vi "Multirecord Acquisition (FPGA)_20221208.vi"() -> ()   [LabVIEW 2021]
doc: "Use this VI as a template for the reconfigurable oscilloscope acquisition design. The block diagram is divided into three main loops.\n\nRegister Bus: This loop initializes the registers that are needed to support the configuration of the device. The FIFO bus, on the left, allows all the other design libraries to communicate with one another. This loop is very important to support the proper behavior of the instrument design library components.\n\nAcquisition: Acquires data from the I/O channels and writes the data into the record memory using the <B>Write</B> VI of the Multirecord Acquisition instrument design library. This VI also evaluates the various acquisition triggers and decides whether to acquire each data value in record memory. The host level VI (Fetch Record.vi) can read acquired records from the DRAM. The data is stored in 2 DRAM banks, each with 768 MB of storage.\n\nFetch: The recorded data is retrieved when the <B>Fetch Single Record</B> VI is run from the host VI. The <B>Write to Fetch DMA FIFO</B> VI writes data to the acq.fetch fifo 0 to transmit record data form the FPGA to the record fetch VIs on the host. This DMA FIFO must have a predefined name based on the instance parameter. By default, it is 0 (since the associated terminal on the <B>Create Resources DRAM Write Read</B> VI is unwired), so the connected FIFO is named acq.fetch fifo 0."
uses:
  FPGA Interface Typedefinitions/Trigger Combination Type.ctl
  <instrlib>/_niInstr/Data Trigger/v1/Shared/Public/Level Configuration FXP(+-,18,1).ctl
  <instrlib>/_niInstr/Data Trigger/v1/Shared/Public/Level Configuration Trigger When.ctl
  <vilib>/Platform/TimedLoop/XDataNode/timing_clust.ctl
  <vilib>/Platform/TimedLoop/XDataNode/nitl_modes.ctl
  <vilib>/Platform/TimedLoop/XDataNode/wakeup.ctl
  <instrlib>/_niInstr/FIFO Register Bus/v1/FPGA/niInstr FIFO Register Bus v1 FPGA.lvclass
  C:/Program Files (x86)/National Instruments/LabVIEW 2021/instr.lib/_niInstr/Instruction Framework/v1/FPGA/Interfaces/Instruction Producer/Instruction Producer.lvclass
  <instrlib>/_niInstr/Multirecord Acquisition/Common/v1/FPGA/niInstr Multirecord Acquisition Common v1 FPGA.lvclass
  C:/Program Files (x86)/National Instruments/LabVIEW 2021/instr.lib/_niInstr/Multirecord Acquisition/Interface/v1/FPGA/niInstr Multirecord Acquisition v1 FPGA.lvclass
  <vilib>/rvi/Emulation/niFpgaSctlEmulationGetInTimedLoop.vi
  <vilib>/rvi/Emulation/niFpgaEmulationReportErrorSimple.vi
  <vilib>/rvi/Emulation/niFpgaGetClockAttributes.vi
  <vilib>/rvi/Emulation/niFpgaCriticalErrorInLSC.vi
  <instrlib>/_niInstr/Multirecord Acquisition/Common/v1/FPGA/Private/Create Fetch DMA FIFO Resources U8x32.vi
  <instrlib>/_niInstr/Multirecord Acquisition/Common/v1/FPGA/Private/Create Resources DRAM U384x2 U768 Write Read.vi
  <instrlib>/_niInstr/Multirecord Acquisition/Interface/v1/FPGA/Private/Retrieve Record U16 Wrapper.vi
  <instrlib>/_niInstr/Multirecord Acquisition/Interface/v1/FPGA/Private/Write to Fetch DMA FIFO U16 Wrapper.vi
  <vilib>/rvi/eio/common/nirviEmuTemplateMethod_errors.vi
  <instrlib>/HSAI-RIO/Config/Group A/v1/FPGA/Digital Correction/Validate 8 Channel Data.vi
  <instrlib>/HSAI-RIO/Config/Group A/v1/FPGA/Digital Correction/Digital Correction (8 Ch).vi
  <instrlib>/HSAI-RIO/Config/Group A/v1/FPGA/Digital Correction/FIR Filter (8 Ch).vi
  DSP/SubVIs/Integer decimationx8ch.vi
  Data Type Conversion/SubVIs/Remove Overflow FXP(+-,18,1)x8ch.vi
  <instrlib>/_niInstr/Channel/v1/FPGA/Private/Select/Select FXP(+-,18,1,)xNspcx8ch.vi
  Trigger/Trigger FXP(+,-,18,1).vi
  Data Type Conversion/SubVIs/Data Type Conversion FXP(+-,18,1) to I16x8ch.vi
  <instrlib>/_niInstr/Channel/v1/FPGA/Private/Select and Interleave/Select And Interleave I16xNspcx8ch.vi
  <instrlib>/_niInstr/Multirecord Acquisition/Interface/v1/FPGA/Private/Write I16 Wrapper.vi
  <vilib>/Platform/TimedLoop/XDataNode/XDataNode.xnode
  <vilib>/eio/EIONode/EIONode.xnode
  <instrlib>/_niInstr/Instruction Framework/v1/FPGA/Top Level Bus/Register Configuration/Register Configuration.lvclass
  <vilib>/Platform/TimedLoop/XDataNode/XDNodeRunTimeDep.lvlib
  <instrlib>/_niInstr/Multirecord Acquisition/Interface/v1/FPGA/niInstr Multirecord Acquisition v1 FPGA.lvclass
  <vilib>/rvi/LocalResourceManager/LocalResourceManager.xnode
  <vilib>/rvi/eio/common/nirviEmuReportErrorAndStop.vi
  <vilib>/rvi/DataTransferAndStorage/Container/Common/niFpgaContainerGetUniqueNameForEmu.vi
  <vilib>/rvi/DataTransferAndStorage/Container/Common/niFpgaContainerSetEmuInfo.vi
  <instrlib>/_niInstr/Channel/v1/FPGA/niInstr Channel v1 FPGA.lvlib
  <instrlib>/_niInstr/Basic Elements/v1/FPGA/niInstr Basic Elements v1 FPGA.lvlib
  <instrlib>/HSAI-RIO/Config/Group A/v1/FPGA/Digital Correction/Digital Correction.lvclass
  <instrlib>/HSAI-RIO/Config/Group A/v1/FPGA/Config Registers/Config Registers.lvclass
  <instrlib>/_niInstr/Multirecord Acquisition/Common/v1/FPGA/Private/Create Resources BRAM U384.vi
  Emulation/SubVIs/2 Element Generate Sine Cos Data FXP(+,-,14,1).vi
  <instrlib>/_niInstr/Multirecord Acquisition/Common/v1/FPGA/Private/Create Resources DRAM U384.vi
  <instrlib>/_niInstr/Multirecord Acquisition/Common/v1/FPGA/Private/Create Resources BRAM U768.vi
  C:/Program Files (x86)/National Instruments/LabVIEW 2021/instr.lib/_niInstr/Multirecord Acquisition/Common/v1/FPGA/niInstr Multirecord Acquisition Common v1 FPGA.lvclass
  FPGA Interface Typedefinitions/FPGA Interface Typedefinitions.lvlib
  <instrlib>/_niInstr/Data Trigger/v1/Shared/niInstr Data Trigger v1 Shared.lvlib
panel:
  in  "trig 7":cluster{"Hi":T1, "Lo":T1}
  in  "trig 6":cluster{"Hi":T1, "Lo":T1}
  in  "trig 5":cluster{"Hi":T1, "Lo":T1}
  in  "trig 4":cluster{"Hi":T1, "Lo":T1}
  in  "trig 3":cluster{"Hi":T1, "Lo":T1}
  in  "trig 2":cluster{"Hi":T1, "Lo":T1}
  in  "trig 1":cluster{"Hi":T1, "Lo":T1}
  in  "trig 0":cluster{"Hi":T1, "Lo":T1}
  in  "trigger.rearm delay":u16=2
  in  "start trigger":bool=TRUE
  in  "reset":bool
  in  "trigger.combination type":T3
  out "fifo reg bus data 0":u64
  out "fifo reg bus status 0":u32
  in  "fifo reg bus ctrl 0":u32
  out "overflow":bool
  in  "dsp.decimation factor":u16
  out "overload":bool
  in  "channel.enable mask":u16=65535 format="%.0b"
  in  "channel.number of channels":u8=8
  # "Register Bus Controls"
  # "FPGA"
  # "Acquisition Loop Controls"
  # "DSP"
  # "Trigger"
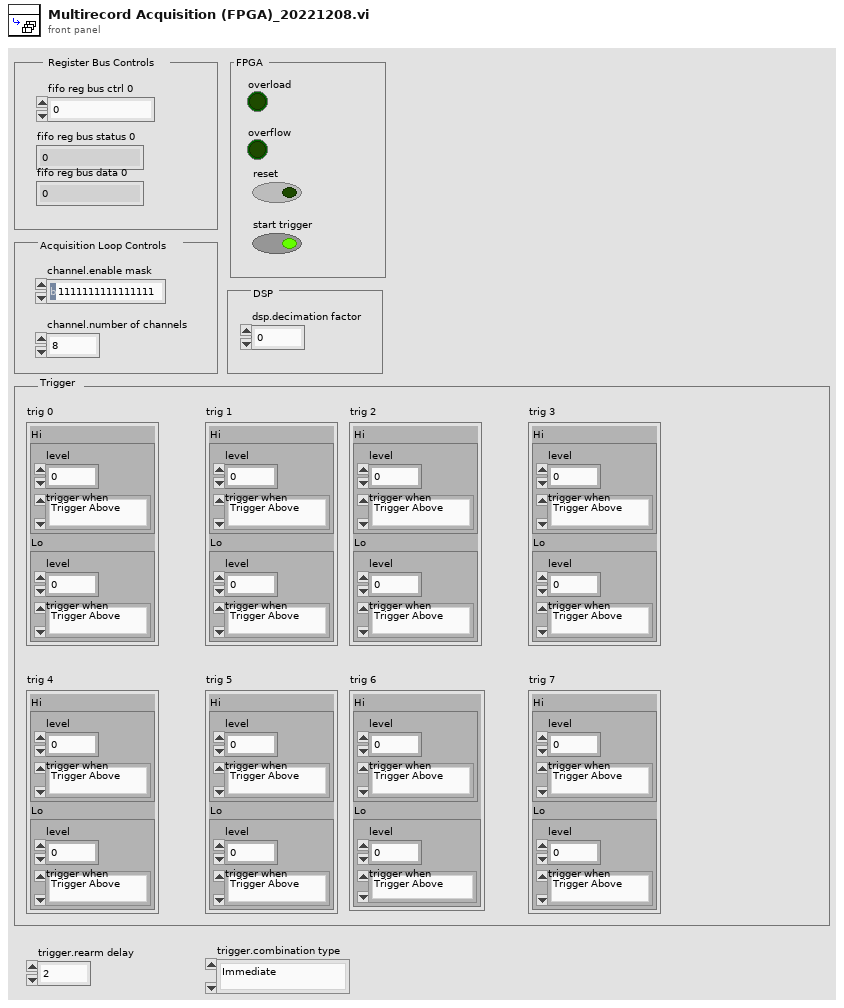
[diagram p1: front panel]
types:
  T1 = typedef "niInstr Data Trigger v1 Shared.lvlib/Level Configuration FXP(+-,18,1).ctl" = cluster{"level":fxp<+/-,18,1>, "trigger when":T2}
  T2 = typedef "niInstr Data Trigger v1 Shared.lvlib/Level Configuration Trigger When.ctl" = enum8{"Trigger Above", "Trigger Below"}
  T3 = typedef "FPGA Interface Typedefinitions.lvlib/Trigger Combination Type.ctl" = enum16{"Immediate", "A", "B", "OR", "AND", "A THEN B", "B THEN A", "High Resolution"}
  T4 = cluster{"memory 1":refnum<k21>, "memory 2":refnum<k21>}
  T5 = typedef "XDNodeRunTimeDep.lvlib/timing_clust.ctl" = cluster{"Expected End [f-1]":u64, "Actual End [f-1]":u64, "Finished Late? [f-1]":bool, "Expected End [i-1]":u64, "Actual End [i-1]":u64, "Finished Late? [i-1]":bool, "Expected Start [i]":u64, "Actual Start [i]":u64, "Expected Start [f]":u64, "Actual Start [f]":u64, "Source Name":string, "Structure Name":string, "Period":i64, "Deadline":i64, "Offset":i64, "Start":i64, "Priority":i32, "Timeout":i32, "Mode":T6, "Wakeup Reason":T7, "Error":errorcluster, "Source Type":string, "Secondary Source Type":string, "Global End Time":u64, "Global Start Time":u64, "Frame Duration":u64, "Iteration Duration":u64, "Assigned CPU":i32, "I/O Scan Engine Mode":u32}
  T6 = typedef "XDNodeRunTimeDep.lvlib/nitl_modes.ctl" = enum32{"No Change", "Process missed periods, maintain original phase", "Discard missed periods, maintain original phase", "Process missed periods, ignore original phase", "Discard missed periods, ignore original phase"}
  T7 = typedef "XDNodeRunTimeDep.lvlib/wakeup.ctl" = enum32{"Normal", "Aborted", "Asynchronous wakeup", "Timing source error", "Timed loop error", "Timeout"}
  T8 = cluster{"Channel 0":fxp<+/-,14,1>[], "Channel 1":fxp<+/-,14,1>[], "Channel 2":fxp<+/-,14,1>[], "Channel 3":fxp<+/-,14,1>[], "Channel 4":fxp<+/-,14,1>[], "Channel 5":fxp<+/-,14,1>[], "Channel 6":fxp<+/-,14,1>[], "Channel 7":fxp<+/-,14,1>[]}
  T9 = cluster{"Channel 0":fxp<+/-,18,1>[], "Channel 1":fxp<+/-,18,1>[], "Channel 2":fxp<+/-,18,1>[], "Channel 3":fxp<+/-,18,1>[], "Channel 4":fxp<+/-,18,1>[], "Channel 5":fxp<+/-,18,1>[], "Channel 6":fxp<+/-,18,1>[], "Channel 7":fxp<+/-,18,1>[]}
  T10 = cluster{"channel 0":fxp<+/-,18,1>[], "channel 1":fxp<+/-,18,1>[], "channel 2":fxp<+/-,18,1>[], "channel 3":fxp<+/-,18,1>[], "channel 4":fxp<+/-,18,1>[], "channel 5":fxp<+/-,18,1>[], "channel 6":fxp<+/-,18,1>[], "channel 7":fxp<+/-,18,1>[]}
  T11 = cluster{"channel 0":i16[], "channel 1":i16[], "channel 2":i16[], "channel 3":i16[], "channel 4":i16[], "channel 5":i16[], "channel 6":i16[], "channel 7":i16[]}
  T12 = typedef "niInstr Multirecord Acquisition v1 FPGA.lvclass/Timestamp.ctl" = cluster{"timestamp":u64, "valid":bool}
  T13 = typedef "niInstr Types v1 Shared.lvlib/Input Triggers.ctl" = cluster{"start":bool, "advance":bool, "reference":bool, "start trigger index":u16, "advance trigger index":u16, "reference trigger index":u16, "reference trigger correction cycle count":u32}
  T14 = typedef "niInstr Types v1 Shared.lvlib/Sample Format.ctl" = cluster{"bits per channel":u16, "samples per clock":u16, "channels":u8}
  T15 = typedef "niInstr Multirecord Acquisition v1 FPGA.lvclass/Events.ctl" = cluster{"ready for start":bool, "ready for advance":bool, "ready for reference":bool, "end of record":bool, "done":bool, "start trigger":bool, "advance trigger":bool, "reference trigger":bool, "start trigger index":u16, "advance trigger index":u16, "reference trigger index":u16}
  T16 = typedef "niInstr Multirecord Acquisition v1 FPGA.lvclass/Retrieve Data Info.ctl" = cluster{"read request size (bits)":u64, "valid data offset (bits)":u16, "valid data size (bits)":u16, "first sample of request":bool, "last sample of request":bool, "Token":T17}
  T17 = typedef "niInstr Types v1 Shared.lvlib/Token.ctl" = cluster{"identifier":u8, "value":u32}
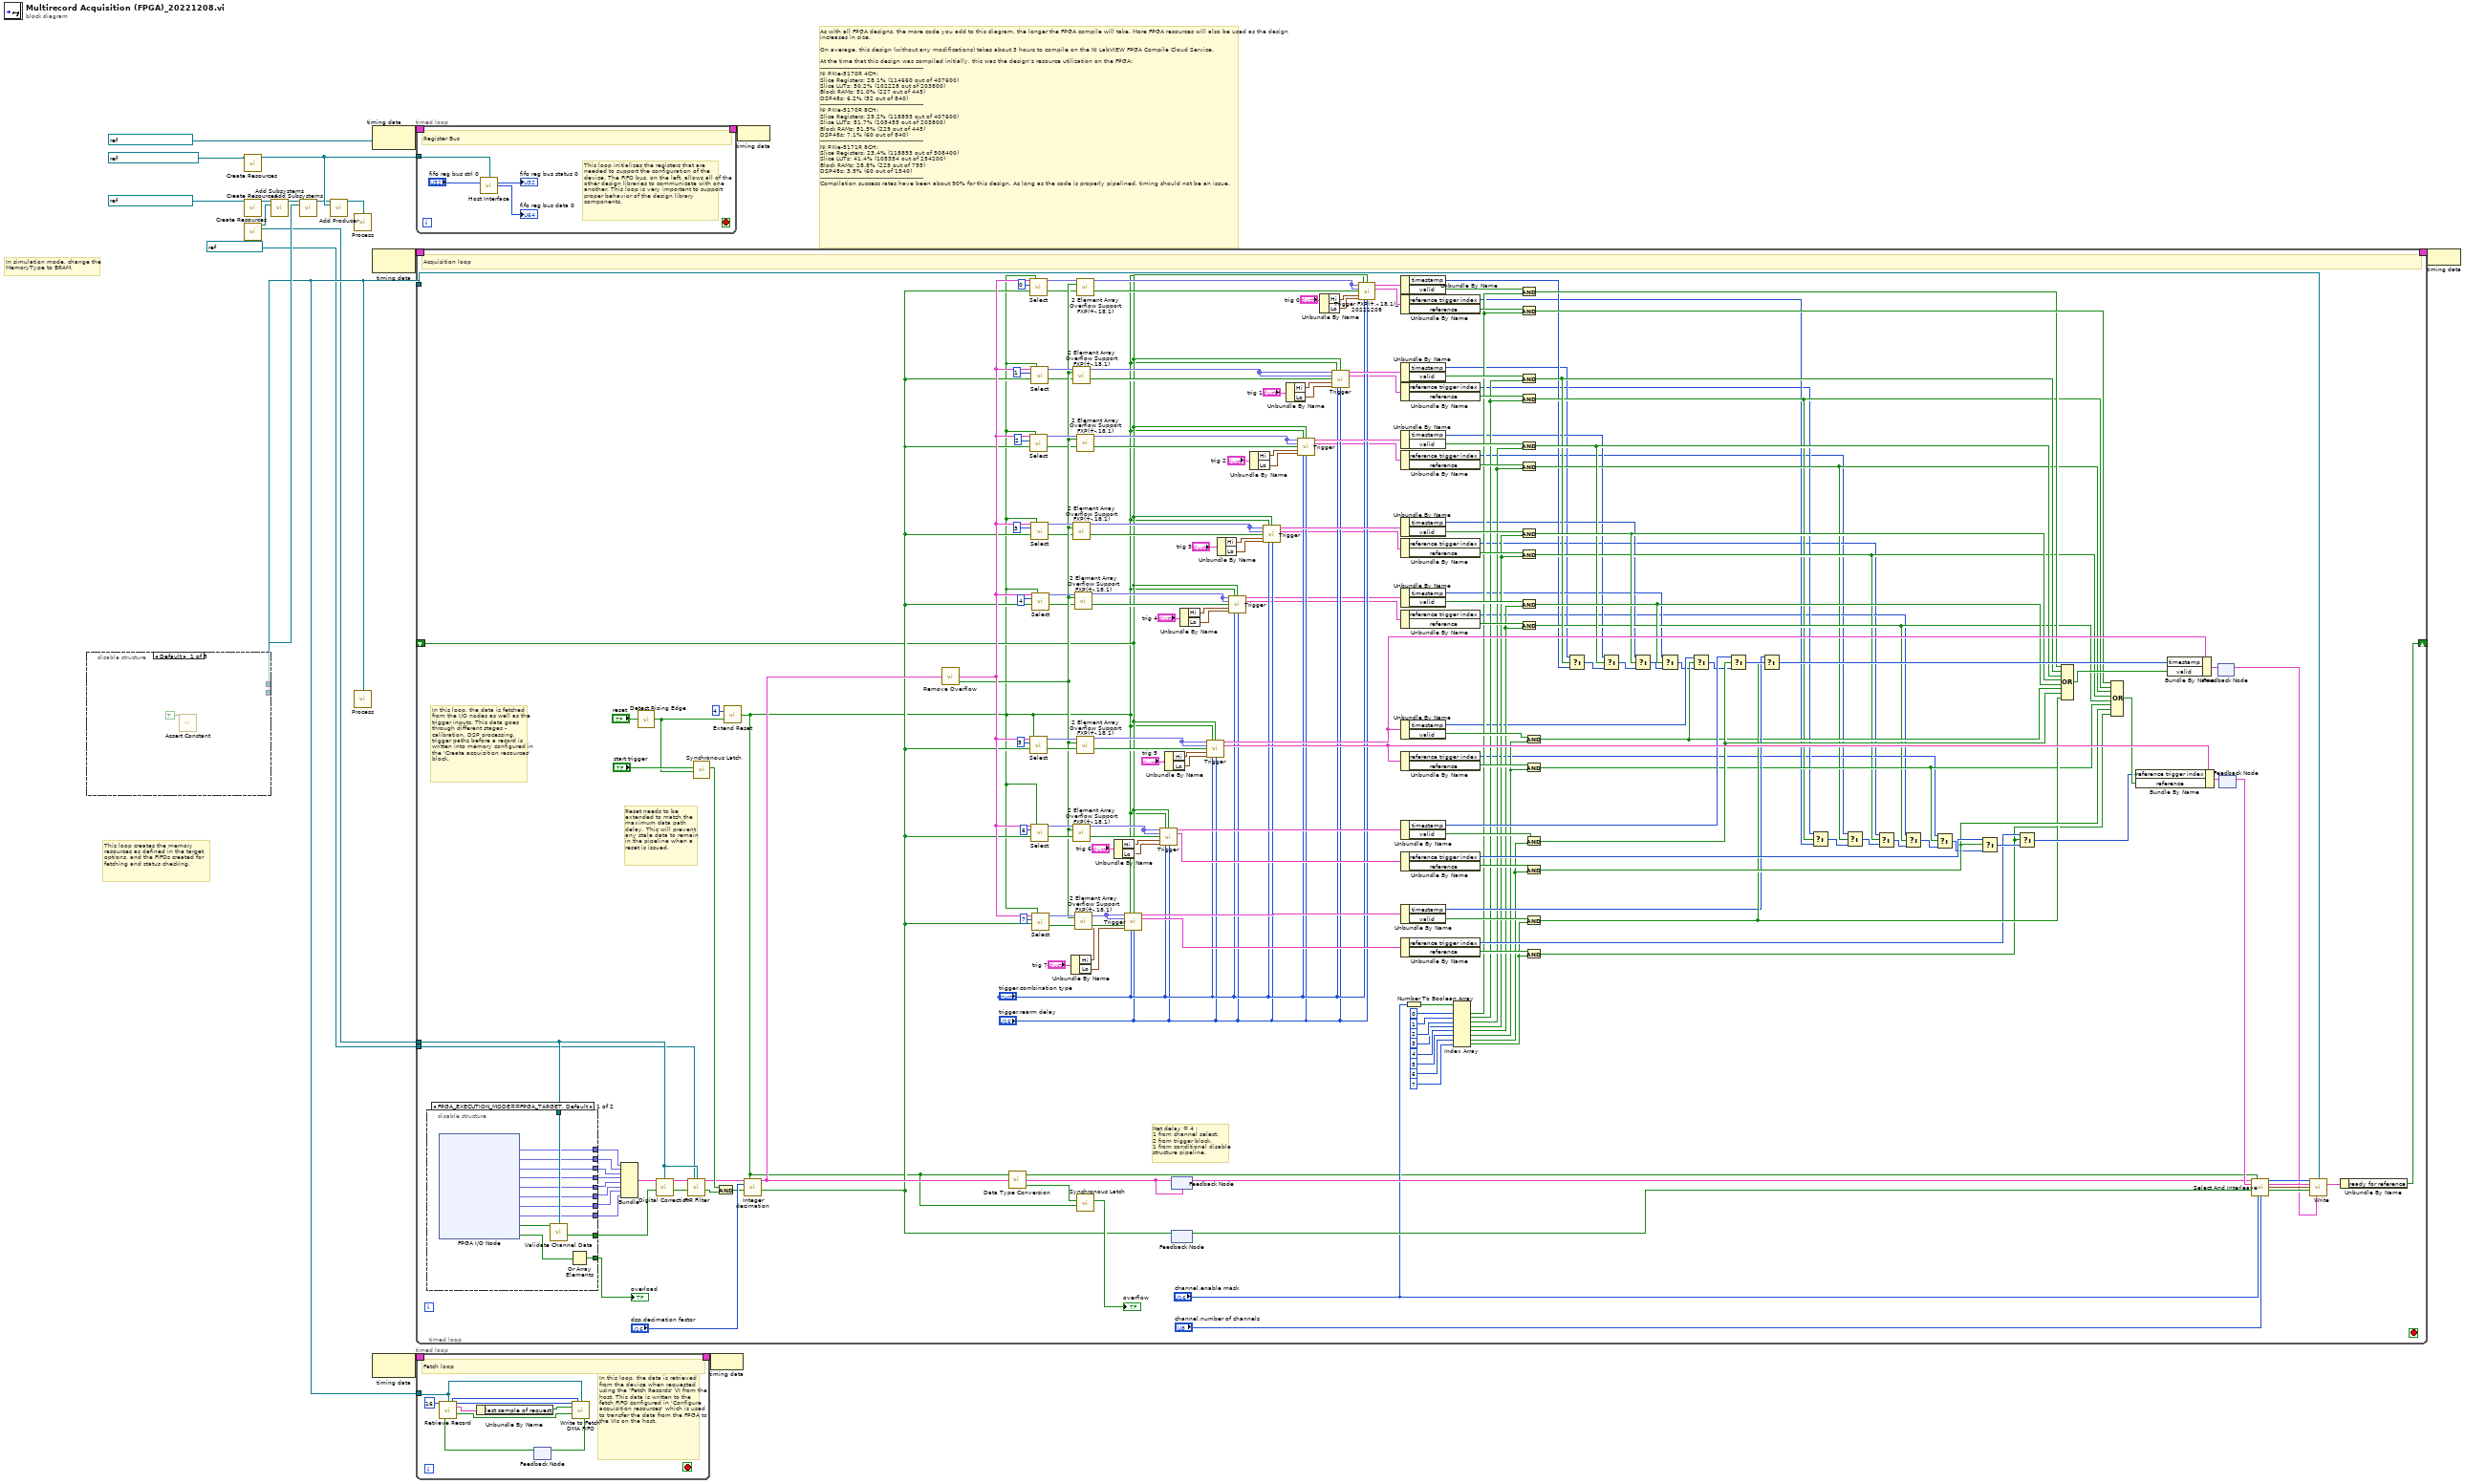
[diagram p0: block diagram]
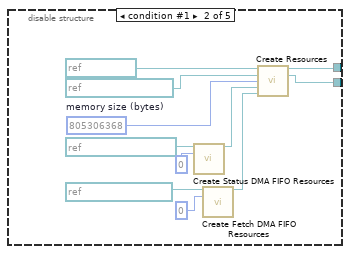
[diagram p2: hidden frame]
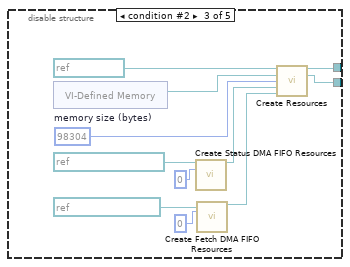
[diagram p3: hidden frame]
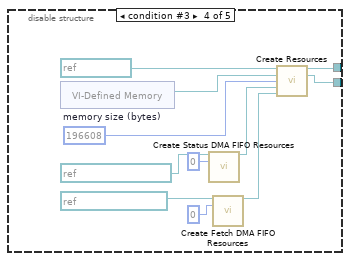
[diagram p4: hidden frame]
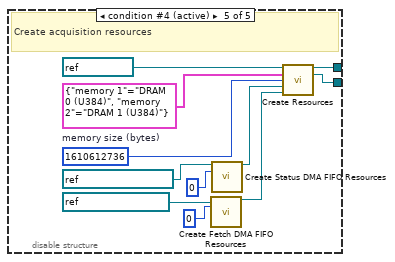
[diagram p5: hidden frame]
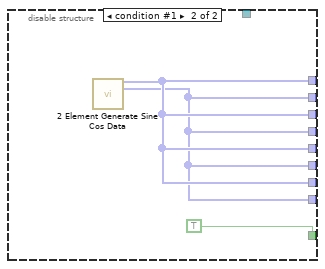
[diagram p6: hidden frame]
diagram:
  # "In simulation mode, change the MemoryType to BRAM."
  # "This loop creates the memory resources as defined in the target options, and the FIFOs created for fetching and status checking."
  # "As with all FPGA designs, the more code you add to this diagram, the longer the FPGA compile will take. More FPGA resources will also be used as the design increases in size.\n\nOn average, this design (without any modifications) takes about 3 hours to compile on the NI LabVIEW FPGA Compile Cloud Service. \n\nAt the time that this design was compiled initially, this was the design's resource utilization on the FPGA:\n------------------------------------------------------\nNI PXIe-5170R 4CH:\nSlice Registers: 28.1% (114660 out of 407600)\nSlice LUTs: 50.2% (102228 out of 203800)\nBlock RAMs: 51.0% (227 out of 445)\nDSP48s: 6.2% (52 out of 840)\n------------------------------------------------------\nNI PXIe-5170R 8CH:\nSlice Registers: 29.2% (118893 out of 407600)\nSlice LUTs: 51.7% (105455 out of 203800)\nBlock RAMs: 51.5% (229 out of 445)\nDSP48s: 7.1% (60 out of 840)\n------------------------------------------------------\nNI PXIe-5171R 8CH:\nSlice Registers: 23.4% (118893 out of 508400)\nSlice LUTs: 41.4% (105354 out of 254200)\nBlock RAMs: 28.8% (229 out of 795)\nDSP48s: 3.9% (60 out of 1540)\n------------------------------------------------------\nCompilation success rates have been about 90% for this design. As long as the code is properly pipelined, timing should not be an issue."
  n1 = disable-structure shown="Default" {
    disable-tunnel: [_ w29 w40 w51 w62] -> w4
    disable-tunnel: [_ w26 w36 w47 w59] -> w7
    frame condition #0 {
      n2 = call <instrlib>:"Assert Constant.vi"("constant terminal"=TRUE) -> ()  [unwired: 15 in]
    }
    frame condition #1 {
      w30 = u64 805306368  # memory size (bytes)
      n3 = call <instrlib>:"Create Status DMA FIFO Resources.vi"("status dma fifo in"=refnum<k21> "acq.status fifo 0" ("status dma fifo"), "fifo instance"=u8 0) -> ("status dma fifo out"=w21:refnum<class "niInstr Status FIFO v1 FPGA.lvclass">)  [unwired: 13 in]
      n4 = call-poly <instrlib>:"Create Fetch DMA FIFO Resources.vi"("fetch dma fifo in"=refnum<k21> "acq.fetch fifo 0", "fifo instance"=u8 0) -> ("fetch dma fifo out"=w27:refnum<class "niInstr Fetch FIFO v1 FPGA.lvclass">)  [unwired: 13 in]
      n5 = call-poly <instrlib>:"Create Resources.vi"("memory clock"=refnum<k21> "160MHz" ("process clock"), "memory"=refnum<k21> "DRAM 0 (U384)" ("dram"), "memory size (bytes)"=w30, "status dma fifo resources"=w21, "fetch dma fifo resources"=w27) -> ("acquisition resources"=w29:refnum<class "niInstr Multirecord Acquisition Common v1 FPGA.lvclass">, "acquisition subsystem"=w26:refnum<class "Address Space Collection.lvclass">)  [unwired: 9 in]
    }
    frame condition #2 {
      w41 = u64 98304  # memory size (bytes)
      n6 = xnode "VI-Defined Memory"() -> ("Memory Out"=w42:refnum<k21>)
      n7 = call <instrlib>:"Create Status DMA FIFO Resources.vi"("status dma fifo in"=refnum<k21> "acq.status fifo 0" ("status dma fifo"), "fifo instance"=u8 0) -> ("status dma fifo out"=w33:refnum<class "niInstr Status FIFO v1 FPGA.lvclass">)  [unwired: 13 in]
      n8 = call-poly <instrlib>:"Create Fetch DMA FIFO Resources.vi"("fetch dma fifo in"=refnum<k21> "acq.fetch fifo 0", "fifo instance"=u8 0) -> ("fetch dma fifo out"=w37:refnum<class "niInstr Fetch FIFO v1 FPGA.lvclass">)  [unwired: 13 in]
      n9 = call-poly <instrlib>:"Create Resources.vi"("memory clock"=refnum<k21> "160MHz" ("process clock"), "memory"=w42, "memory size (bytes)"=w41, "status dma fifo resources"=w33, "fetch dma fifo resources"=w37) -> ("acquisition resources"=w40:refnum<class "niInstr Multirecord Acquisition Common v1 FPGA.lvclass">, "acquisition subsystem"=w36:refnum<class "Address Space Collection.lvclass">)  [unwired: 9 in]
    }
    frame condition #3 {
      w52 = u64 196608  # memory size (bytes)
      n10 = xnode "VI-Defined Memory"() -> ("Memory Out"=w53:refnum<k21>)
      n11 = call <instrlib>:"Create Status DMA FIFO Resources.vi"("status dma fifo in"=refnum<k21> "acq.status fifo 0" ("status dma fifo"), "fifo instance"=u8 0) -> ("status dma fifo out"=w45:refnum<class "niInstr Status FIFO v1 FPGA.lvclass">)  [unwired: 13 in]
      n12 = call-poly <instrlib>:"Create Fetch DMA FIFO Resources.vi"("fetch dma fifo in"=refnum<k21> "acq.fetch fifo 0", "fifo instance"=u8 0) -> ("fetch dma fifo out"=w48:refnum<class "niInstr Fetch FIFO v1 FPGA.lvclass">)  [unwired: 13 in]
      n13 = call-poly <instrlib>:"Create Resources.vi"("memory clock"=refnum<k21> "160MHz" ("process clock"), "memory"=w53, "memory size (bytes)"=w52, "status dma fifo resources"=w45, "fetch dma fifo resources"=w48) -> ("acquisition resources"=w51:refnum<class "niInstr Multirecord Acquisition Common v1 FPGA.lvclass">, "acquisition subsystem"=w47:refnum<class "Address Space Collection.lvclass">)  [unwired: 9 in]
    }
    frame condition #4 (active) {
      w64 = u64 1610612736  # memory size (bytes)
      # "Create acquisition resources"
      n14 = call-poly <instrlib>:"Create Fetch DMA FIFO Resources.vi"("fetch dma fifo in"=refnum<k21> "acq.fetch fifo 0", "fifo instance"=u8 0) -> ("fetch dma fifo out"=w61:refnum<class "niInstr Fetch FIFO v1 FPGA.lvclass">)  [unwired: 13 in]
      n15 = call <instrlib>:"Create Status DMA FIFO Resources.vi"("status dma fifo in"=refnum<k21> "acq.status fifo 0" ("status dma fifo"), "fifo instance"=u8 0) -> ("status dma fifo out"=w56:refnum<class "niInstr Status FIFO v1 FPGA.lvclass">)  [unwired: 13 in]
      n16 = call-poly <instrlib>:"Create Resources.vi"("memory clock"=refnum<k21> "160MHz" ("process clock"), "memory"=T4 {"memory 1"="DRAM 0 (U384)", "memory 2"="DRAM 1 (U384)"}, "memory size (bytes)"=w64, "status dma fifo resources"=w56, "fetch dma fifo resources"=w61) -> ("acquisition resources"=w62:refnum<class "niInstr Multirecord Acquisition Common v1 FPGA.lvclass">, "acquisition subsystem"=w59:refnum<class "Address Space Collection.lvclass">)  [unwired: 9 in]
    }
  }
  n17 = call <instrlib>:"Create Resources.vi"("instruction fifo"=refnum<k21> "reg.host instruction fifo 0" ("FIFO")) -> ("fifo register bus"=w6:refnum<class "niInstr FIFO Register Bus v1 FPGA.lvclass">)  [unwired: 14 in]
  n18 = call <instrlib>:"Create Resources.vi"("register clock"=refnum<k21> "40 MHz Onboard Clock" ("Source Name")) -> ("register configuration"=w10:refnum<class "Register Configuration.lvclass">)  [unwired: 14 in]
  n19 = call <instrlib>:"Create Resources.vi"() -> ("config subsystems"=w8:refnum<class "Address Space Collection.lvclass">, "digital correction resources"=w1:refnum<class "Digital Correction.lvclass">)  [unwired: 14 in]
  n20 = call-dynamic "Add Subsystems.vi"("register configuration in"=w10, "subsystems"=w8) -> ("register configuration out"=w9:refnum<class "Register Configuration.lvclass">)  [unwired: 13 in]
  n21 = call-dynamic "Add Subsystems.vi"("register configuration in"=w9, "subsystems"=w7) -> ("register configuration out"=w3:refnum<class "Register Configuration.lvclass">)  [unwired: 13 in]
  n22 = call-dynamic "Add Producer.vi"("register configuration in"=w3, "instruction producer"=w6) -> ("register configuration out"=w5:refnum<class "Register Configuration.lvclass">)  [unwired: 13 in]
  n23 = call-dynamic "Process.vi"("register configuration"=w5) -> ()  [unwired: 15 in]
  n24 = call-dynamic "Process.vi"("acquisition resources"=w4) -> ()  [unwired: 15 in]
  n25 = node-c288(refnum<k21> "40 MHz Onboard Clock" ("Source Name")) -> (w19:T5)
  n26 = node-c288() -> (w17:T5)  [unwired: 1 in]
  n27 = node-c288() -> (w15:T5)  [unwired: 1 in]
  n28 = timed-loop {
    timing: w19 -> [_]
    timing-out: [_] -> w18
    tunnel: w6 -> [w68]
    stop <- _ stop-if-true
    # "This loop initializes the registers that are needed to support the configuration of the device. The FIFO bus, on the left, allows all of the other design libraries to communicate with one another. This loop is very important to support proper behavior of the design library components."
    # "Register Bus"
    n29 = call <instrlib>:"Host Interface.vi"("fifo register bus"=w68, "fifo reg bus ctrl 0"="fifo reg bus ctrl 0") -> ("fifo reg bus status 0"=→"fifo reg bus status 0":u32, "fifo reg bus data 0"=→"fifo reg bus data 0":u64)  [unwired: 12 in]
  }
  n30 = timed-loop {
    timing: w17 -> [_]
    timing-out: [_] -> w16
    tunnel: w4 -> [w272]
    tunnel: w1 -> [w255]
    shift-right: [w264] -> _
    shift-left: _ -> [w167]
    tunnel: refnum<k21> "Data Clock x2" -> [w252]
    stop <- _ stop-if-true
    # "Net delay = 4 :\n1 from channel select.\n2 from trigger block.\n1 from conditional disable structure pipeline."
    # "Reset needs to be extended to match the maximum data path delay. This will prevent any stale data to remain in the pipeline when a reset is issued."
    # "In this loop, the data is fetched from the I/O nodes as well as the trigger inputs. This data goes through different stages - calibration, DSP processing, trigger paths before a record is written into memory configured in the 'Create acquisition resources' block."
    # "Acquisition loop"
    n31 = disable-structure shown="FPGA_EXECUTION_MODE==FPGA_TARGET, Default" {
      disable-tunnel: [w284 w289] -> w251
      disable-tunnel: [w283 w288] -> w250
      disable-tunnel: [w282 w289] -> w249
      disable-tunnel: [w281 w288] -> w248
      disable-tunnel: [w280 w289] -> w247
      disable-tunnel: [w279 w288] -> w246
      disable-tunnel: [w278 w289] -> w244
      disable-tunnel: [w277 w288] -> w245
      disable-tunnel: [w274 TRUE ("ADC Data Valid")] -> w242
      disable-tunnel: w255 -> [w285 _]
      disable-tunnel: [w275 _] -> w271
      frame condition #0 (active) {
        # "I/O Nodes"
        n32 = xnode "FPGA I/O Node"() -> ("Channel 0"=w284:fxp<+/-,14,1>[], "Channel 1"=w283:fxp<+/-,14,1>[], "Channel 2"=w282:fxp<+/-,14,1>[], "Channel 3"=w281:fxp<+/-,14,1>[], "Channel 4"=w280:fxp<+/-,14,1>[], "Channel 5"=w279:fxp<+/-,14,1>[], "Channel 6"=w278:fxp<+/-,14,1>[], "Channel 7"=w277:fxp<+/-,14,1>[], "Channel Data Valid"=w286:bool[], "Channel Overload"=w276:bool[])  [unwired: 10 in, 10 out]
        n33 = call-poly <instrlib>:"Validate Channel Data.vi"("channel data valid"=w286, "digital correction resources"=w285) -> ("expected data valid"=w274:bool)  [unwired: 13 in]
        n34 = Or Array Elements(Boolean array=w276) -> (logical OR=w275:bool)
      }
      frame condition #1 {
        n35 = call-poly "2 Element Generate Sine Cos Data.vi"() -> ("sine data"=w289:fxp<+/-,14,1>[], "cosine data"=w288:fxp<+/-,14,1>[])  [unwired: 14 in]
      }
    }
    "overload" <- w271
    n36 = Bundle("Channel 0"=w251, "Channel 1"=w250, "Channel 2"=w249, "Channel 3"=w248, "Channel 4"=w247, "Channel 5"=w246, "Channel 6"=w244, "Channel 7"=w245) -> (w243:T8)  [unwired: 1 in]
    n37 = call <instrlib>:"Detect Rising Edge.vi"("signal"="reset") -> ("edge detected"=w254:bool)  [unwired: 14 in]
    n38 = call-poly <instrlib>:"Digital Correction.vi"("channel data in"=w243, "digital correction resources"=w255, "input valid"=w242) -> ("corrected channel data out"=w235:T9, "output valid"=w234:bool)  [unwired: 11 in]
    n39 = call-poly <instrlib>:"FIR Filter.vi"("data in"=w235, "data clock x2"=w252, "digital correction resources"=w255, "input valid"=w234) -> ("data out"=w232:T9, "output valid"=w233:bool)  [unwired: 9 in, 1 out]
    n40 = call <instrlib>:"Synchronous Latch.vi"("clear"=w254, "set"="start trigger") -> ("out"=w260:bool)  [unwired: 9 in]
    n41 = And(x=w260, y=w233) -> (x .and. y?=w236:bool)
    n42 = call "Extend Reset.vi"("reset in"=w254, "number of cycles"=u8 4) -> ("reset out"=w71:bool)
    n43 = call-poly "Integer decimation.vi"("data in"=w232, "reset"=w71, "decimation factor"="dsp.decimation factor", "input valid"=w236) -> ("data out"=w239:T10, "output valid"=w183:bool)  [unwired: 9 in, 1 out]
    n44 = call-poly "Remove Overflow.vi"("data in"=w239) -> ("overflow"=w177:bool, "data out"=w189:T10)  [unwired: 3 in]
    n45 = call-poly "Data Type Conversion.vi"("data in"=w239) -> ("overflow"=w241:bool, "data out"=w238:T11)  [unwired: 3 in]
    n46 = call-poly <instrlib>:"Select.vi"("data in"=w189, "reset"=w71, "channel index"=u8 0 ("trigger.channel A"), "input valid"=w183) -> ("channel out"=w188:fxp<+/-,18,1>[], "output valid"=w172:bool)  [unwired: 10 in]
    n47 = call-poly <instrlib>:"Select.vi"("data in"=w189, "reset"=w71, "channel index"=u8 2 ("trigger.channel A"), "input valid"=w183) -> ("channel out"=w186:fxp<+/-,18,1>[], "output valid"=w174:bool)  [unwired: 10 in]
    n48 = call-poly <instrlib>:"Select.vi"("data in"=w189, "reset"=w71, "channel index"=u8 5 ("trigger.channel A"), "input valid"=w183) -> ("channel out"=w262:fxp<+/-,18,1>[], "output valid"=w231:bool)  [unwired: 10 in]
    n49 = call-poly <instrlib>:"Select.vi"("data in"=w189, "reset"=w71, "channel index"=u8 1, "input valid"=w183) -> ("channel out"=w187:fxp<+/-,18,1>[], "output valid"=w173:bool)  [unwired: 10 in]
    n50 = call-poly <instrlib>:"Select.vi"("data in"=w189, "reset"=w71, "channel index"=u8 3, "input valid"=w183) -> ("channel out"=w185:fxp<+/-,18,1>[], "output valid"=w175:bool)  [unwired: 10 in]
    n51 = call-poly <instrlib>:"Select.vi"("data in"=w189, "reset"=w71, "channel index"=u8 6, "input valid"=w183) -> ("channel out"=w228:fxp<+/-,18,1>[], "output valid"=w226:bool)  [unwired: 10 in]
    n52 = call-poly <instrlib>:"Select.vi"("data in"=w189, "reset"=w71, "channel index"=u8 4, "input valid"=w183) -> ("channel out"=w184:fxp<+/-,18,1>[], "output valid"=w176:bool)  [unwired: 10 in]
    n53 = call-poly <instrlib>:"Select.vi"("data in"=w189, "reset"=w71, "channel index"=u8 7, "input valid"=w183) -> ("channel out"=w207:fxp<+/-,18,1>[], "output valid"=w205:bool)  [unwired: 10 in]
    n54 = Unbundle By Name("trig 7") -> ("Hi"=w73:T1, "Lo"=w72:T1)
    n55 = call "2 Element Array Overflow Support FXP(+-,18,1).vi"("data in"=w187, "overflow"=w177) -> ("data out"=w181:fxp<+/-,18,1>[])  [unwired: 13 in]
    n56 = call "2 Element Array Overflow Support FXP(+-,18,1).vi"("data in"=w185, "overflow"=w177) -> ("data out"=w179:fxp<+/-,18,1>[])  [unwired: 13 in]
    n57 = call "2 Element Array Overflow Support FXP(+-,18,1).vi"("data in"=w228, "overflow"=w177) -> ("data out"=w227:fxp<+/-,18,1>[])  [unwired: 13 in]
    n58 = call "2 Element Array Overflow Support FXP(+-,18,1).vi"("data in"=w184, "overflow"=w177) -> ("data out"=w178:fxp<+/-,18,1>[])  [unwired: 13 in]
    n59 = call "2 Element Array Overflow Support FXP(+-,18,1).vi"("data in"=w207, "overflow"=w177) -> ("data out"=w206:fxp<+/-,18,1>[])  [unwired: 13 in]
    n60 = call "2 Element Array Overflow Support FXP(+-,18,1).vi"("data in"=w188, "overflow"=w177) -> ("data out"=w182:fxp<+/-,18,1>[])  [unwired: 13 in]
    n61 = call "2 Element Array Overflow Support FXP(+-,18,1).vi"("data in"=w186, "overflow"=w177) -> ("data out"=w180:fxp<+/-,18,1>[])  [unwired: 13 in]
    n62 = call "2 Element Array Overflow Support FXP(+-,18,1).vi"("data in"=w262, "overflow"=w177) -> ("data out"=w230:fxp<+/-,18,1>[])  [unwired: 13 in]
    n63 = call <instrlib>:"Synchronous Latch.vi"("clear"=w71, "set"=w241) -> ("out"=→"overflow":bool)  [unwired: 9 in]
    n64 = Unbundle By Name("trig 6") -> ("Hi"=w76:T1, "Lo"=w75:T1)
    n65 = call-poly "Trigger.vi"("data A"=w206, "reset"=w71, "trigger.ready for reference"=w167, "data B"=w206, "input valid"=w205, "trigger.level Hi"=w73, "trigger.level Lo"=w72, "trigger.combination type"="trigger.combination type", "rearm delay"="trigger.rearm delay") -> ("timestamps"=w204:T12, "trigger.out"=w203:T13)  [unwired: 4 in, 1 out]
    n66 = call-poly "Trigger.vi"("data A"=w227, "reset"=w71, "trigger.ready for reference"=w167, "data B"=w227, "input valid"=w226, "trigger.level Hi"=w76, "trigger.level Lo"=w75, "trigger.combination type"="trigger.combination type", "rearm delay"="trigger.rearm delay") -> ("timestamps"=w221:T12, "trigger.out"=w220:T13)  [unwired: 4 in, 1 out]
    n67 = Unbundle By Name("trig 5") -> ("Hi"=w79:T1, "Lo"=w78:T1)
    n68 = feedback #1(w238) -> (w240:T11)
    n69 = feedback-in #1(w238) -> ()
    n70 = feedback #2() -> (w237:bool)  [unwired: 1 in]
    n71 = feedback-in #2(w183) -> ()
    n72 = Unbundle By Name("trig 4") -> ("Hi"=w82:T1, "Lo"=w81:T1)
    n73 = call-poly "Trigger.vi"("data A"=w230, "reset"=w71, "trigger.ready for reference"=w167, "data B"=w230, "input valid"=w231, "trigger.level Hi"=w79, "trigger.level Lo"=w78, "trigger.combination type"="trigger.combination type", "rearm delay"="trigger.rearm delay") -> ("timestamps"=w225:T12, "trigger.out"=w223:T13)  [unwired: 4 in, 1 out]
    n74 = Unbundle By Name("trig 3") -> ("Hi"=w85:T1, "Lo"=w84:T1)
    n75 = call-poly "Trigger.vi"("data A"=w178, "reset"=w71, "trigger.ready for reference"=w167, "data B"=w178, "input valid"=w176, "trigger.level Hi"=w82, "trigger.level Lo"=w81, "trigger.combination type"="trigger.combination type", "rearm delay"="trigger.rearm delay") -> ("timestamps"=w160:T12, "trigger.out"=w159:T13)  [unwired: 4 in, 1 out]
    n76 = Unbundle By Name("trig 2") -> ("Hi"=w88:T1, "Lo"=w87:T1)
    n77 = call-poly "Trigger.vi"("data A"=w179, "reset"=w71, "trigger.ready for reference"=w167, "data B"=w179, "input valid"=w175, "trigger.level Hi"=w85, "trigger.level Lo"=w84, "trigger.combination type"="trigger.combination type", "rearm delay"="trigger.rearm delay") -> ("timestamps"=w168:T12, "trigger.out"=w161:T13)  [unwired: 4 in, 1 out]
    n78 = Unbundle By Name("trig 1") -> ("Hi"=w91:T1, "Lo"=w90:T1)
    n79 = call-poly "Trigger.vi"("data A"=w180, "reset"=w71, "trigger.ready for reference"=w167, "data B"=w180, "input valid"=w174, "trigger.level Hi"=w88, "trigger.level Lo"=w87, "trigger.combination type"="trigger.combination type", "rearm delay"="trigger.rearm delay") -> ("timestamps"=w169:T12, "trigger.out"=w162:T13)  [unwired: 4 in, 1 out]
    n80 = Unbundle By Name("trig 0") -> ("Hi"=w94:T1, "Lo"=w93:T1)
    n81 = call-poly "Trigger.vi"("data A"=w181, "reset"=w71, "trigger.ready for reference"=w167, "data B"=w181, "input valid"=w173, "trigger.level Hi"=w91, "trigger.level Lo"=w90, "trigger.combination type"="trigger.combination type", "rearm delay"="trigger.rearm delay") -> ("timestamps"=w170:T12, "trigger.out"=w163:T13)  [unwired: 4 in, 1 out]
    n82 = call "Trigger FXP(+,-,18,1)_20221208.vi"("data A"=w182, "reset"=w71, "trigger.ready for reference"=w167, "data B"=w182, "input valid"=w172, "trigger.level Hi"=w94, "trigger.level Lo"=w93, "trigger.combination type"="trigger.combination type", "rearm delay"="trigger.rearm delay") -> ("timestamps"=w171:T12, "trigger.out"=w164:T13)  [unwired: 4 in, 1 out]
    n83 = Unbundle By Name(w171) -> ("timestamp"=w122:u64, "valid"=w153:bool)
    n84 = Unbundle By Name(w164) -> ("reference trigger index"=w111:u16, "reference"=w152:bool)
    n85 = Unbundle By Name(w170) -> ("timestamp"=w112:u64, "valid"=w151:bool)
    n86 = Unbundle By Name(w163) -> ("reference trigger index"=w110:u16, "reference"=w150:bool)
    n87 = Unbundle By Name(w169) -> ("timestamp"=w113:u64, "valid"=w149:bool)
    n88 = Unbundle By Name(w162) -> ("reference trigger index"=w101:u16, "reference"=w148:bool)
    n89 = Unbundle By Name(w168) -> ("timestamp"=w114:u64, "valid"=w147:bool)
    n90 = Unbundle By Name(w161) -> ("reference trigger index"=w102:u16, "reference"=w146:bool)
    n91 = Unbundle By Name(w160) -> ("timestamp"=w115:u64, "valid"=w145:bool)
    n92 = Unbundle By Name(w159) -> ("reference trigger index"=w103:u16, "reference"=w144:bool)
    n93 = Unbundle By Name(w225) -> ("timestamp"=w121:u64, "valid"=w213:bool)
    n94 = Unbundle By Name(w223) -> ("reference trigger index"=w105:u16, "reference"=w211:bool)
    n95 = Unbundle By Name(w221) -> ("timestamp"=w219:u64, "valid"=w212:bool)
    n96 = Unbundle By Name(w220) -> ("reference trigger index"=w218:u16, "reference"=w210:bool)
    n97 = Unbundle By Name(w204) -> ("timestamp"=w191:u64, "valid"=w201:bool)
    n98 = Unbundle By Name(w203) -> ("reference trigger index"=w190:u16, "reference"=w202:bool)
    n99 = Number To Boolean Array(number="channel.enable mask") -> (Boolean array=w216:bool[])
    n100 = Index Array(array=w216, index #1=0 ("index"), index #2=1 ("index"), index #3=2 ("index"), index #4=3 ("index"), index #5=4 ("index"), index #6=5 ("index"), index #7=6 ("index"), index #8=7 ("index")) -> (element #1=w143:bool, element #2=w142:bool, element #3=w141:bool, element #4=w140:bool, element #5=w139:bool, element #6=w138:bool, element #7=w137:bool, element #8=w136:bool)
    n101 = And(x=w153, y=w143) -> (x .and. y?=w133:bool)
    n102 = And(x=w152, y=w143) -> (x .and. y?=w134:bool)
    n103 = And(x=w151, y=w142) -> (x .and. y?=w128:bool)
    n104 = And(x=w150, y=w142) -> (x .and. y?=w123:bool)
    n105 = And(x=w149, y=w141) -> (x .and. y?=w129:bool)
    n106 = And(x=w148, y=w141) -> (x .and. y?=w124:bool)
    n107 = And(x=w147, y=w140) -> (x .and. y?=w130:bool)
    n108 = And(x=w146, y=w140) -> (x .and. y?=w125:bool)
    n109 = And(x=w145, y=w139) -> (x .and. y?=w131:bool)
    n110 = And(x=w144, y=w139) -> (x .and. y?=w126:bool)
    n111 = And(x=w213, y=w138) -> (x .and. y?=w132:bool)
    n112 = And(x=w211, y=w138) -> (x .and. y?=w127:bool)
    n113 = And(x=w212, y=w137) -> (x .and. y?=w200:bool)
    n114 = And(x=w210, y=w137) -> (x .and. y?=w198:bool)
    n115 = And(x=w201, y=w136) -> (x .and. y?=w192:bool)
    n116 = And(x=w202, y=w136) -> (x .and. y?=w135:bool)
    n117 = Select(t=w112, s=w128, f=w122) -> (s? t:f=w116:u64)
    n118 = Select(t=w113, s=w129, f=w116) -> (s? t:f=w117:u64)
    n119 = Select(t=w114, s=w130, f=w117) -> (s? t:f=w118:u64)
    n120 = Select(t=w115, s=w131, f=w118) -> (s? t:f=w119:u64)
    n121 = Select(t=w121, s=w132, f=w119) -> (s? t:f=w120:u64)
    n122 = Select(t=w219, s=w200, f=w120) -> (s? t:f=w196:u64)
    n123 = Select(t=w191, s=w192, f=w196) -> (s? t:f=w195:u64)
    n124 = Select(t=w110, s=w123, f=w111) -> (s? t:f=w109:u16)
    n125 = Select(t=w101, s=w124, f=w109) -> (s? t:f=w108:u16)
    n126 = Select(t=w102, s=w125, f=w108) -> (s? t:f=w107:u16)
    n127 = Select(t=w103, s=w126, f=w107) -> (s? t:f=w106:u16)
    n128 = Select(t=w105, s=w127, f=w106) -> (s? t:f=w104:u16)
    n129 = Select(t=w218, s=w198, f=w104) -> (s? t:f=w194:u16)
    n130 = Select(t=w190, s=w135, f=w194) -> (s? t:f=w193:u16)
    n131 = Compound Arithmetic op=OR(w133, w128, w129, w130, w131, w132, w200, w192) -> (w199:bool)
    n132 = Compound Arithmetic op=OR(w134, w123, w124, w125, w126, w127, w198, w135) -> (w197:bool)
    n133 = Bundle By Name(cluster=w223, "reference trigger index"=w193, "reference"=w197) -> (w222:T13)
    n134 = Bundle By Name(cluster=w225, "timestamp"=w195, "valid"=w199) -> (w224:T12)
    n135 = feedback #3() -> (w258:T12)  [unwired: 1 in]
    n136 = feedback-in #3(w224) -> ()
    n137 = feedback #4() -> (w259:T13)  [unwired: 1 in]
    n138 = feedback-in #4(w222) -> ()
    n139 = call-poly <instrlib>:"Select And Interleave.vi"("data in"=w240, "reset"=w71, "triggers in"=w259, "input valid"=w237, "channel enable mask"="channel.enable mask", "number of channels to interleave"="channel.number of channels") -> ("interleaved data out"=w270:i16[], "triggers out"=w269:T13, "sample format out"=w268:T14, "output valid"=w267:bool)  [unwired: 5 in, 1 out]
    n140 = call-poly <instrlib>:"Write.vi"("data"=w270, "acquisition resources"=w272, "triggers"=w269, "sample format"=w268, "data valid"=w267, "timestamp"=w258) -> ("events"=w265:T15)  [unwired: 7 in, 2 out]
    n141 = Unbundle By Name(w265) -> ("ready for reference"=w264:bool)
  }
  n142 = timed-loop {
    timing: w15 -> [_]
    timing-out: [_] -> w14
    tunnel: w4 -> [w300]
    stop <- _ stop-if-true
    # "In this loop, the data is retrieved from the device when requested using the 'Fetch Records' VI from the host. This data is written to the fetch FIFO configured in 'Configure acquisition resources' which is used to transfer the data from the FPGA to the VIs on the host."
    # "Fetch loop"
    n143 = feedback #5() -> (w298:bool)  [unwired: 1 in]
    n144 = call-poly <instrlib>:"Retrieve Record.vi"("output array size"=u16 16, "acquisition resources"=w300, "ready for output"=w298) -> ("channels"=w293:u8, "data"=w296:u16[], "retrieve data info"=w295:T16, "output valid"=w297:bool)  [unwired: 9 in]
    n145 = Unbundle By Name(w295) -> ("last sample of request"=w294:bool)
    n146 = call-poly <instrlib>:"Write to Fetch DMA FIFO.vi"("data"=w296, "channels"=w293, "acquisition resources"=w300, "last sample of request"=w294, "input valid"=w297) -> ("ready for input"=w299:bool)  [unwired: 10 in]
    n147 = feedback-in #5(w299) -> ()
  }
  n148 = node-c288(w14) -> ()
  n149 = node-c288(w18) -> ()
  n150 = node-c288(w16) -> ()
